vi "Manager Camera Communication.vi"(8 "error in (no error)":errorcluster, 11 "Channel in":refnum<class "Channel.lvclass">) -> (0 "error out":errorcluster, 3 "Channel out":refnum<class "Channel.lvclass">)   [LabVIEW 2018, in "Channel.lvclass"]
uses:
  Channel.lvclass
  Channel.lvclass/Channel.ctl
  Simulated_CCD_Camera/Simulated_CCD_Camera.lvclass/Simulated_CCD_Camera.ctl
  State Machine/State Machine.lvclass/State Machine.ctl
  Interface/Interface.lvclass
  State Machine/State Machine.lvclass
  Simulated_CCD_Camera/Simulated_CCD_Camera.lvclass
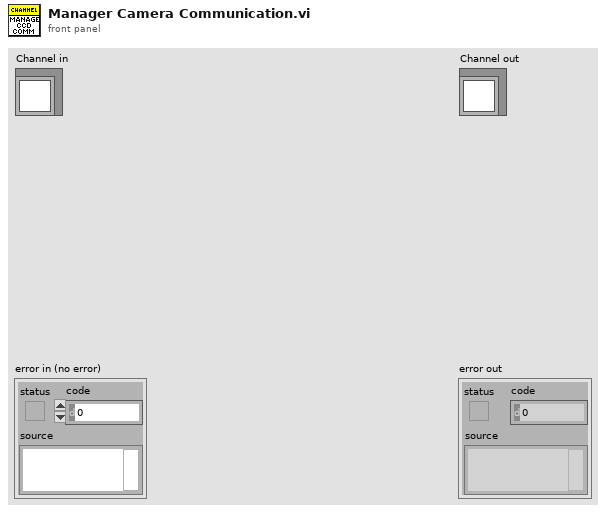
[diagram p1: front panel]
types:
  T1 = cluster{"CUBE_EXPOSURE_TIME":sgl, "CUBES_DONE":u16, "LAST_IMAGE_NAME":string, "DISK_SPACE":u16, "FRAMES_DONE":u16, "CCD_STATUS":string, "CURRENT_TEMPERATURE":i16, "TEMPERATURE_STATUS":string, "FRAME_EXPOSURE_TIME":u16, "CCD_ON_OFF":bool, "SERIAL_NUMBER":u16, "ACQUIRING":bool}
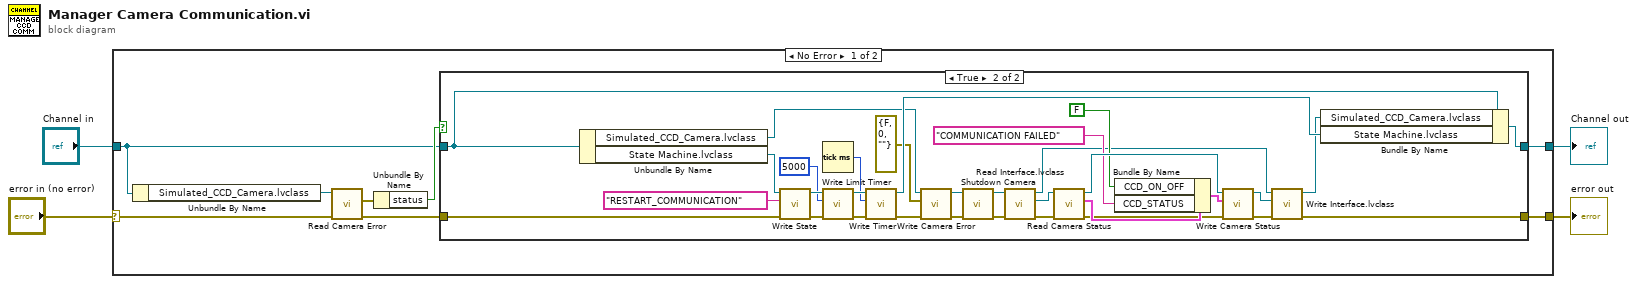
[diagram p0: block diagram]
diagram:
  n1 = case shown="No Error" "error in (no error)" {
    selector: "error in (no error)" -> [w12 w48]
    tunnel: [w7 w48] -> w3
    tunnel: [w6 w47] -> w1
    tunnel: "Channel in" -> [w9 w47]
    frame No Error {
      n2 = Unbundle By Name(w9) -> ("Simulated_CCD_Camera.lvclass"=w5:refnum<class "Simulated_CCD_Camera.lvclass">)
      n3 = call "Read Camera Error.vi"("error in (no error)"=w12, "Simulated_CCD_Camera in"=w5) -> ("error out"=w8:errorcluster, "Camera Error"=w11:errorcluster)  [unwired: 7 in, 1 out]
      n4 = Unbundle By Name(w11) -> ("status"=w10:bool)
      n5 = case shown="True" w10 {
        tunnel: w9 -> [w14 w33]
        tunnel: w8 -> [w13 w45]
        tunnel: [w13 w32] -> w7
        tunnel: [w14 w31] -> w6
        frame False {
        }
        frame True {
          n6 = Unbundle By Name(w33) -> ("Simulated_CCD_Camera.lvclass"=w15:refnum<class "Simulated_CCD_Camera.lvclass">, "State Machine.lvclass"=w46:refnum<class "State Machine.lvclass">)
          n7 = call-dynamic "Write State.vi"("error in (no error)"=w45, "State"="RESTART_COMMUNICATION" ("CCD_STATUS"), "State Machine in"=w46) -> ("error out"=w28:errorcluster, "State Machine out"=w29:refnum<class "State Machine.lvclass">)  [unwired: 7 in]
          n8 = Tick Count (ms)() -> (millisecond timer value=w21:u32)
          n9 = call "Write Limit Timer.vi"("error in (no error)"=w28, "Limit Timer"=u32 5000, "State Machine in"=w29) -> ("error out"=w23:errorcluster, "State Machine out"=w24:refnum<class "State Machine.lvclass">)  [unwired: 7 in]
          n10 = call "Write Timer.vi"("error in (no error)"=w23, "Timer"=w21, "State Machine in"=w24) -> ("error out"=w16:errorcluster, "State Machine out"=w22:refnum<class "State Machine.lvclass">)  [unwired: 7 in]
          n11 = call "Write Camera Error.vi"("error in (no error)"=w16, "Camera Error"=errorcluster {"status"=FALSE, "code"=0, "source"=""}, "Simulated_CCD_Camera in"=w15) -> ("error out"=w19:errorcluster, "Simulated_CCD_Camera out"=w20:refnum<class "Simulated_CCD_Camera.lvclass">)  [unwired: 7 in]
          n12 = call-dynamic "Shutdown Camera.vi"("error in (no error)"=w19, "CCDCamera in"=w20) -> ("error out"=w25:errorcluster, "CCDCamera out"=w26:refnum<class "Simulated_CCD_Camera.lvclass">)  [unwired: 8 in]
          n13 = call "Read Interface.lvclass.vi"("error in (no error)"=w25, "Simulated_CCD_Camera in"=w26) -> ("error out"=w42:errorcluster, "Interface.lvclass"=w43:refnum<class "Interface.lvclass">, "Simulated_CCD_Camera out"=w34:refnum<class "Simulated_CCD_Camera.lvclass">)  [unwired: 7 in]
          n14 = call "Read Camera Status.vi"("error in (no error)"=w42, "Interface in"=w43) -> ("error out"=w41:errorcluster, "Camera Status"=w44:T1, "Interface out"=w39:refnum<class "Interface.lvclass">)  [unwired: 7 in]
          n15 = Bundle By Name(cluster=w44, "CCD_ON_OFF"=FALSE, "CCD_STATUS"="COMMUNICATION FAILED") -> (w40:T1)
          n16 = call "Write Camera Status.vi"("error in (no error)"=w41, "Camera Status"=w40, "Interface in"=w39) -> ("error out"=w35:errorcluster, "Interface out"=w36:refnum<class "Interface.lvclass">)  [unwired: 7 in]
          n17 = call "Write Interface.lvclass.vi"("error in (no error)"=w35, "Interface.lvclass"=w36, "Simulated_CCD_Camera in"=w34) -> ("error out"=w32:errorcluster, "Simulated_CCD_Camera out"=w17:refnum<class "Simulated_CCD_Camera.lvclass">)  [unwired: 7 in]
          n18 = Bundle By Name(cluster=w33, "Simulated_CCD_Camera.lvclass"=w17, "State Machine.lvclass"=w22) -> (w31:refnum<class "Channel.lvclass">)
        }
      }
    }
    frame Error {
    }
  }
  "error out" <- w3
  "Channel out" <- w1
